vi "Set Query.vi"(8 "error in (no error)":errorcluster, 10 "Query":string, 11 "URI in":refnum<class "URI.lvclass">) -> (0 "error out":errorcluster, 3 "URI out":refnum<class "URI.lvclass">)   [LabVIEW 2020, in "Stream.lvlib" / "URI.lvclass"]
uses:
  URI.lvclass
  URI.lvclass/URI.ctl
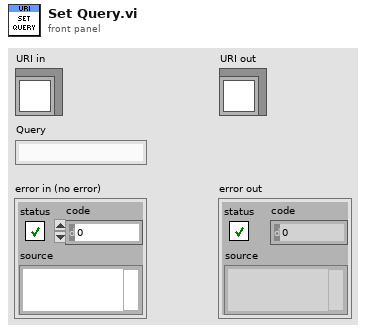
[diagram p1: front panel]
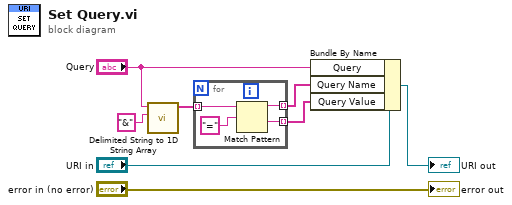
[diagram p0: block diagram]
diagram:
  n1 = call <vilib>:"Delimited String to 1D String Array.vi"("delimiter"="&", "delimited string"="Query") -> ("string array"=w3:string[])  [unwired: 9 in]
  n2 = for {
    tunnel: w3 -> [w12] mode=indexing
    tunnel: [w10] -> w5 mode=indexing
    tunnel: [w9] -> w4 mode=indexing
    n3 = Match Pattern(string=w12, regular expression="=") -> (before substring=w10:string, after substring=w9:string)  [unwired: 1 in, 2 out]
  }
  n4 = Bundle By Name(cluster="URI in", "Query"="Query", "Query Name"=w5, "Query Value"=w4) -> (→"URI out":refnum<class "URI.lvclass">)
  "error out" <- "error in (no error)"
